vi "Query Count Display.vi"(8 "error in (no error)":errorcluster, 9 "Read B?":bool, 11 "VISA resource name":refnum<visa-resource-name>) -> (0 "error out":errorcluster, 1 "Counts":dbl, 3 "VISA resource name out":refnum<visa-resource-name>)   [LabVIEW 2015, in "SR400.lvlib"]
uses:
  SR400.lvlib
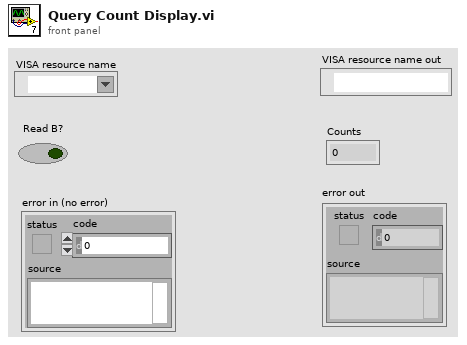
[diagram p1: front panel]
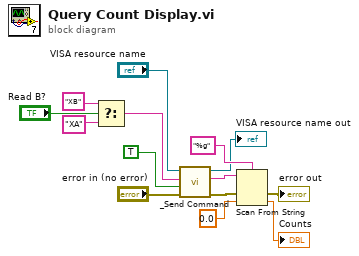
[diagram p0: block diagram]
diagram:
  n1 = Select(t="XB" ("command"), s="Read B?", f="XA" ("command")) -> (s? t:f=w6:string)
  n2 = call "_Send Command.vi"("error in (no error)"="error in (no error)", "Query? (F)"=TRUE, "Command"=w6, "VISA resource name"="VISA resource name") -> ("error out"=w2:errorcluster, "Response"=w3:string, "VISA resource name out"=→"VISA resource name out":refnum<visa-resource-name>)  [unwired: 5 out]
  n3 = Scan From String(format string="%g", input string=w3, error in=w2, default 1=0.0 ("default value 1")) -> (error out=→"error out":errorcluster, output 1=→"Counts":dbl)  [unwired: 1 in, 2 out]
